vi "Nested Malleable VIs - Lesson 1.vi"() -> ()   [LabVIEW 2023]
doc: "Lesson 1 discusses how nesting malleable VIs can solve the problem of trying to keep two Type Specialization structures in sync."
uses:
  70628e59-3872-47d4-8fe0-9b1cb31e2cbd.vi
  194a96a1-6648-4a15-af4e-2eab6c2abee7.vi
  e407c2ba-2cdc-4439-b839-37b982fad3e3.vi
  5db0d465-61b2-4d19-833d-5bf5f7303d5f.vi
  72ee5810-4f74-4d7c-91cf-ebcb76086e83.vi
  41e33179-9614-409c-ace5-27ca9a350ff8.vi
  70628e59-3872-47d4-8fe0-9b1cb31e2cbd.vi/4bbec9e6-ad34-4531-be30-7e5514c76a12.vi
  194a96a1-6648-4a15-af4e-2eab6c2abee7.vi/49c810e3-b63b-4e87-b49c-019c015d9d6d.vi
  72ee5810-4f74-4d7c-91cf-ebcb76086e83.vi/f8e0ef64-138d-4bfd-9277-082e7e533dd8.vi
  41e33179-9614-409c-ace5-27ca9a350ff8.vi/f8e0ef64-138d-4bfd-9277-082e7e533dd8.vi
  35ca6a8b-4785-41e7-904b-10204d6ce6a6.vi
panel:
  in  "Original string 3":string="The quick brown fox jumps over the lazy dog."
  out "Shuffled string 3":string
  in  "Original path 3":path=path "../somewhere/in/the/world/X.vi"
  out "Shuffled path 3":path
  out "shuffled numeric array":i32[](array[numeric])
  in  "Original string 1":string="The quick brown fox jumps over the lazy dog."
  out "Shuffled string 1":string
  in  "Original path 1":path=path "../somewhere/in/the/world/X.vi"
  out "Shuffled path 1":path
  out "Shuffled path 2":path
  in  "Original path 2":path=path "../somewhere/in/the/world/X.vi"
  out "Shuffled string 2":string
  in  "Original string 2":string="The quick brown fox jumps over the lazy dog."
  # "Overview: This example assumes you are familiar with malleable VIs. If you are not, please begin with the examples\\Malleable VIs\\Basics and examples\\Malleable VIs\\Class Adaptaion shipping examples.\n\nThis example shows how you can use nested malleable VIs to create particularly flexible APIs. The particular API demonstrated is for searching and sorting arrays, but the principles apply to many other APIs.\n\nThis first lesson shows a problem that commonly crops up when you want to write a malleable VI: trying to take an existing operation and add code around it.\n\nInstructions: \n1. Open the block diagram of this VI. Review the lessons presented there.\n2. Run the VI to see the results. \n3. Once you have finished reviewing this VI, open the next lesson VI in the Malleable VIs - Nested Malleable VIs example project."
  # "Incorrect solution (does not work right for all types)"
  # "Inefficient solution (works but hard to maintain)"
  # "Recommended solution"
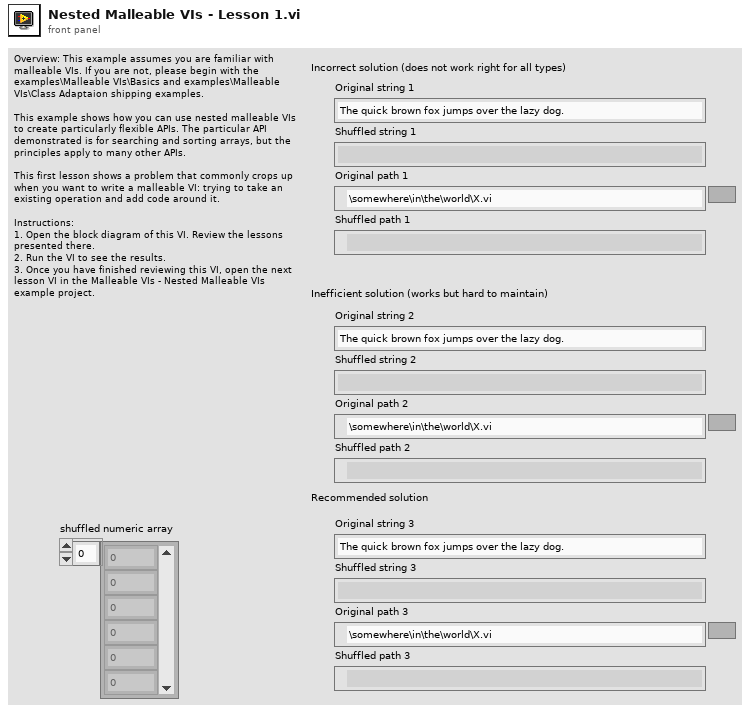
[diagram p1: front panel]
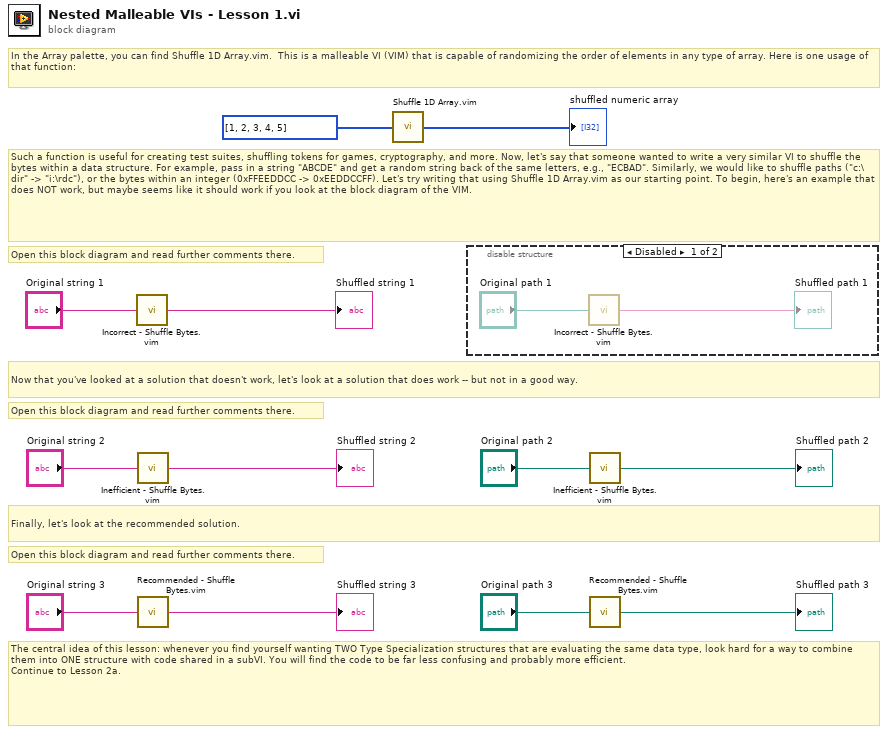
[diagram p0: block diagram]
diagram:
  # "The central idea of this lesson: whenever you find yourself wanting TWO Type Specialization structures that are evaluating the same data type, look hard for a way to combine them into ONE structure with code shared in a subVI. You will find the code to be far less confusing and probably more efficient. \nContinue to Lesson 2a."
  # "Open this block diagram and read further comments there."
  # "Finally, let's look at the recommended solution."
  # "Open this block diagram and read further comments there."
  # "Open this block diagram and read further comments there."
  # "Such a function is useful for creating test suites, shuffling tokens for games, cryptography, and more. Now, let's say that someone wanted to write a very similar VI to shuffle the bytes within a data structure. For example, pass in a string \"ABCDE\" and get a random string back of the same letters, e.g., \"ECBAD\". Similarly, we would like to shuffle paths (\"c:\\dir\" -> \"i:\\rdc\"), or the bytes within an integer (0xFFEEDDCC -> 0xEEDDCCFF). Let's try writing that using Shuffle 1D Array.vim as our starting point. To begin, here's an example that does NOT work, but maybe seems like it should work if you look at the block diagram of the VIM."
  # "In the Array palette, you can find Shuffle 1D Array.vim.  This is a malleable VI (VIM) that is capable of randomizing the order of elements in any type of array. Here is one usage of that function:"
  # "Now that you've looked at a solution that doesn't work, let's look at a solution that does work -- but not in a good way."
  n1 = call "Incorrect - Shuffle Bytes.vim"("original"="Original string 1") -> ("shuffled"=→"Shuffled string 1":string)  [unwired: 4 in]
  n2 = call "Inefficient - Shuffle Bytes.vim"("original"="Original string 2") -> ("shuffled"=→"Shuffled string 2":string)  [unwired: 4 in]
  n3 = call "Recommended - Shuffle Bytes.vim"("original"="Original string 3") -> ("shuffled"=→"Shuffled string 3":string)  [unwired: 4 in]
  n4 = call "Shuffle 1D Array.vim"("array"=i32[] [1, 2, 3, 4, 5]) -> ("shuffled array"=→"shuffled numeric array":i32[])  [unwired: 4 in]
  n5 = disable-structure shown="Disabled" {
    frame Disabled {
      n6 = call "Incorrect - Shuffle Bytes.vim"("original"="Original path 1") -> ("shuffled"=→"Shuffled path 1":string)  [unwired: 4 in]
    }
    frame Enabled {
    }
  }
  n7 = call "Inefficient - Shuffle Bytes.vim"("original"="Original path 2") -> ("shuffled"=→"Shuffled path 2":path)  [unwired: 4 in]
  n8 = call "Recommended - Shuffle Bytes.vim"("original"="Original path 3") -> ("shuffled"=→"Shuffled path 3":path)  [unwired: 4 in]
